vi "Send Enqueuer to Core.vi"(8 "error in (no error)":errorcluster, 10 "Client/Service Enqueuer":refnum<class "Message Enqueuer.lvclass">, 11 "WS Test Client in":refnum<class "WS Client Subscriber.lvclass">) -> (0 "error out":errorcluster, 3 "WS Test Client out":refnum<class "WS Client Subscriber.lvclass">)   [LabVIEW 2021, in "Echo Broadcast With Server Manager.lvlib" / "WS Client Subscriber.lvclass"]
uses:
  WS Client Subscriber.lvclass
  <vilib>/ActorFramework/Message Enqueuer/Message Enqueuer.lvclass
  WS Client Subscriber.lvclass/WS Client Subscriber.ctl
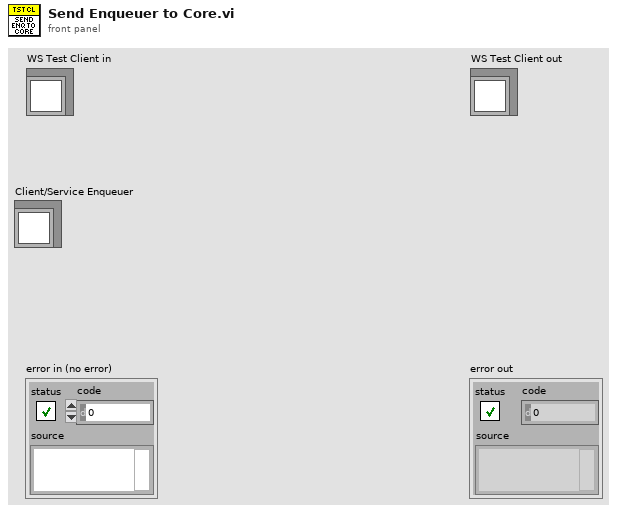
[diagram p1: front panel]
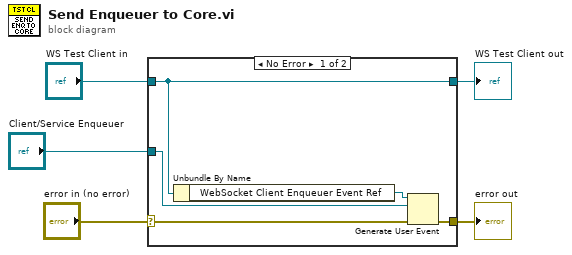
[diagram p0: block diagram]
diagram:
  n1 = case shown="No Error" "error in (no error)" {
    selector: "error in (no error)" -> [w7 w12]
    tunnel: [w6 w12] -> w4
    tunnel: [w10 w11] -> w2
    tunnel: "WS Test Client in" -> [w10 w11]
    tunnel: "Client/Service Enqueuer" -> [w8 _]
    frame No Error {
      n2 = Unbundle By Name(w10) -> ("WebSocket Client Enqueuer Event Ref"=w9:refnum<user-event>)
      n3 = Generate User Event(user event=w9, event data cluster=w8, error in=w7) -> (error out=w6:errorcluster)  [unwired: 1 in, 1 out]
    }
    frame Error {
    }
  }
  "error out" <- w4
  "WS Test Client out" <- w2
